vi "BMU诊断标定.vi"(8 "CAN端口":u16(ring), 9 "设备索引号":u16(ring), 10 "CAN卡类型":u32(ring)=21) -> ()   [LabVIEW 2013] (continued)
    tunnel: w59 -> [w3721]
    tunnel: [w3720] -> w63
    tunnel: [w3719] -> w62
    tunnel: w27 -> [_]
    tunnel: w22 -> [w3711]
    stop <- w3718 stop-if-true
    n2828 = local read "停止"() -> (w3718:bool)
    n2829 = local read "设备索引号"() -> (w3715:u16)
    n2830 = local read "CAN卡类型"() -> (w3716:u32)
    n2831 = local read "CAN端口"() -> (w3714:u16)
    n2832 = call "receiver-8.6.vi"("错误输入（无错误）"=w3711, "CAN端口"=w3714, "设备索引号"=w3715, "CAN卡类型"=w3716) -> ("错误输出"=w3717:errorcluster, "输出簇"=w3713:T25, "接收成功"=w3712:bool)  [unwired: 3 out]
    n2833 = call <vilib>:"Clear Errors.vi"("error in (no error)"=w3717) -> ()  [unwired: 6 in, 1 out]
    n2834 = case shown="真" w3712 {
      tunnel: w3721 -> [w3723 w3729]
      tunnel: w3713 -> [_ w3728]
      tunnel: w3722 -> [w3724 w3727]
      tunnel: [w3724 w3726] -> w3720
      tunnel: [w3723 w3725] -> w3719
      frame False {
      }
      frame True {
        n2835 = Enqueue Element(queue=w3727, element=w3728, error in (no error)=w3729) -> (queue out=w3726:refnum<queue>, error out=w3725:errorcluster)  [unwired: 2 out]
      }
    }
  }
  n2836 = while {
    tunnel: w60 -> [w3739]
    tunnel: w59 -> [w3738]
    tunnel: w8 -> [w3731]
    stop <- w3732 stop-if-true
    n2837 = global read "全局 1.vi" "名称"() -> (w3730:string)
    n2838 = local read "停止"() -> (w3732:bool)
    n2839 = local read "控制1"() -> (w3734:bool)
    n2840 = Dequeue Element(queue=w3739, timeout in ms (-1)=50 ("超时毫秒(-1)"), error in (no error)=w3738) -> (element=w3737:T3, error out=w3736:errorcluster)  [unwired: 2 out]
    n2841 = case shown="无错误" w3736 {
      tunnel: w3737 -> [w3746 _]
      tunnel: "写?" -> [w3743 _]
      tunnel: w3734 -> [w3742 _]
      tunnel: w3731 -> [w3741 _]
      tunnel: w3730 -> [w3740 _]
      frame No Error {
        n2842 = Unbundle(w3746) -> ("return type"=w3745:u32, "pReceive"=w3744:T26)
        n2843 = for {
          N: w3745 -> [_]
          tunnel: w3744 -> [w3752] mode=indexing
          tunnel: w3743 -> [w3750]
          tunnel: w3742 -> [w3749]
          tunnel: w3741 -> [w3748]
          tunnel: w3740 -> [w3747]
          n2844 = Unbundle By Name(w3752) -> ("ID"=w3753:u32)
          n2845 = call "ID解析.vi"("ID"=w3753) -> ("PDU(1)"=w3751:i32)  [unwired: 10 out]
          n2846 = case shown="18" w3751 {
            tunnel: w3752 -> [_ w3765]
            tunnel: w3750 -> [_ w3757]
            tunnel: w3749 -> [_ w3756]
            tunnel: w3748 -> [_ w3755]
            tunnel: w3747 -> [_ w3754]
            frame 0, Default {
            }
            frame 24 {
              n2847 = local read "主从选择"() -> (w3758:enum32{"主板", "从板"})
              n2848 = local read "设备索引号"() -> (w3761:u16)
              n2849 = local read "CAN卡类型"() -> (w3760:u32)
              n2850 = local read "CAN端口"() -> (w3762:u16)
              n2851 = case shown="\"从板\"" w3758 {
                tunnel: [0 ("FUNC") w3768] -> w3759
                tunnel: w3755 -> [_ w3769]
                tunnel: w3754 -> [_ w3767]
                frame "主板", Default {
                }
                frame "从板" {
                  n2852 = local read "从板号"() -> (w3770:u8)
                  n2853 = Equal?(x=w3767, y="从板号") -> (x = y?=w3771:bool)
                  n2854 = Select(t=w3769, s=w3771, f=w3770) -> (s? t:f=w3768:i32)
                }
              }
              n2855 = disable-structure shown="禁用" {
                disable-tunnel: w3765 -> [w3773 _]
                frame Disabled {
                  n2856 = call "标定授权读取.vi"("VCI_Receive"=w3773) -> ()  [unwired: 1 out]
                }
                frame Enabled {
                }
              }
              n2857 = local read "面板选择"() -> (w3764:T7)
              n2858 = case shown="\"读写参数\", 默认" w3764 {
                tunnel: w3757 -> [w3778 _ _ _]
                tunnel: "命令" -> [w3779 w3879 w4134 w4274]
                tunnel: w3758 -> [w3788 _ w4142 w4282]
                tunnel: w3765 -> [_ _ _ _]
                tunnel: w3765 -> [w3784 w3880 w4136 w4276]
                tunnel: w3762 -> [w3783 w3881 w4137 w4277]
                tunnel: w3761 -> [w3782 w3882 w4138 w4278]
                tunnel: w3760 -> [w3781 w3883 w4139 w4279]
                tunnel: w3759 -> [w3780 _ w4135 w4275]
                tunnel: w3756 -> [w3774 _ _ _]
                frame "读写参数", Default {
                  n2859 = local read "命令序号"() -> (w3777:u8)
                  n2860 = call "多帧接收机制(EV05).vi"("can卡类型"=w3781, "设备索引号"=w3782, "CAN端口"=w3783, "VCI_Receive"=w3784, "命令"=w3779, "板号"=w3780, "写?"=w3778, "命令序号"=w3777) -> ("错误信号"=w3775:bool, "错误代码"=w3787:i32, "输出数组"=w3786:u8[], "读错误代码"=w3776:u8[], "结束信号"=w3785:bool)  [unwired: 7 out]
                  n2861 = case shown="假" w3778 {
                    tunnel: w3785 -> [w3798 w3862]
                    tunnel: w3787 -> [w3797 w3861]
                    tunnel: w3777 -> [w3796 _]
                    tunnel: w3786 -> [w3795 _]
                    tunnel: w3779 -> [w3794 _]
                    tunnel: w3788 -> [w3792 w3860]
                    tunnel: w3776 -> [w3791 _]
                    tunnel: w3775 -> [w3790 _]
                    tunnel: w3774 -> [w3789 _]
                    frame False {
                      # "读参数"
                      n2862 = And(x=w3789, y=w3798) -> (x .and. y?=w3793:bool)
                      n2863 = case shown="真" w3793 {
                        tunnel: w3797 -> [_ w3809]
                        tunnel: w3796 -> [_ w3808]
                        tunnel: w3795 -> [_ w3807]
                        tunnel: w3794 -> [_ w3806]
                        tunnel: w3792 -> [_ w3802]
                        tunnel: w3791 -> [_ w3800]
                        tunnel: w3790 -> [_ w3801]
                        frame False {
                        }
                        frame True {
                          n2864 = case shown="假" w3801 {
                            tunnel: w3809 -> [w3819 _]
                            tunnel: w3808 -> [w3818 _]
                            tunnel: w3807 -> [w3817 _]
                            tunnel: w3806 -> [w3815 _]
                            tunnel: w3802 -> [w3811 _]
                            tunnel: w3800 -> [_ w3845]
                            frame False {
                              n2865 = case shown="\"从板\"" w3811 {
                                tunnel: [w3820 _] -> w3814
                                tunnel: [_ w3833] -> w3813
                                frame "主板", Default {
                                n2866 = stacked-sequence {
                                tunnel: [_ w3832] -> w3820
                                frame #0 {
                                n2867 = control-ref of="一级故障"() -> (w3826:refnum<vi>)
                                n2868 = control-ref of="一级故障 2"() -> (w3828:refnum<vi>)
                                n2869 = control-ref of="一级故障 3"() -> (w3829:refnum<vi>)
                                n2870 = control-ref of="加热控制参数"() -> (w3830:refnum<vi>)
                                n2871 = control-ref of="充电控制参数"() -> (w3831:refnum<vi>)
                                n2872 = control-ref of="电池信息"() -> (w3824:refnum<vi>)
                                n2873 = control-ref of="项目信息"() -> (w3827:refnum<vi>)
                                n2874 = control-ref of="项目信息2"() -> (w3825:refnum<vi>)
                                n2875 = control-ref of="高压参数"() -> (w3823:refnum<vi>)
                                n2876 = local read "主板数据"() -> (w3822:T4)
                                n2877 = Bundle(cluster=w3822, "项目信息"=w3827, "一级故障 4"=w3825, "一级故障"=w3826, "一级故障 2"=w3828, "一级故障 3"=w3829, "加热控制参数"=w3830, "充电控制参数"=w3831, "高压参数"=w3823, "电池信息"=w3824) -> (w3821:T4)
                                n2878 = local write "主板数据"(w3821) -> ()
                                }
                                frame #1 {
                                n2879 = control-ref of="主板数据"() -> (w3832:refnum<vi>)
                                }
                                }
                                }
                                frame "从板" {
                                n2880 = stacked-sequence {
                                tunnel: [_ w3844] -> w3833
                                frame #0 {
                                n2881 = control-ref of="从板号"() -> (w3838:refnum<vi>)
                                n2882 = control-ref of="项目信息 2"() -> (w3839:refnum<vi>)
                                n2883 = control-ref of="电池组信息"() -> (w3837:refnum<vi>)
                                n2884 = control-ref of="加热控制参数"() -> (w3840:refnum<vi>)
                                n2885 = control-ref of="一级故障(从板)"() -> (w3841:refnum<vi>)
                                n2886 = control-ref of="二级故障(从板)"() -> (w3842:refnum<vi>)
                                n2887 = control-ref of="三级故障(从板)"() -> (w3843:refnum<vi>)
                                n2888 = control-ref of="均衡参数"() -> (w3836:refnum<vi>)
                                n2889 = local read "从板信息"() -> (w3835:T2)
                                n2890 = Bundle(cluster=w3835, "从板号"=w3838, "项目信息 2"=w3839, "加热控制参数"=w3840, "一级故障(从板)"=w3841, "二级故障(从板)"=w3842, "三级故障(从板)"=w3843, "电池组信息(从板)"=w3837, "均衡参数"=w3836) -> (w3834:T2)
                                n2891 = local write "从板信息"(w3834) -> ()
                                }
                                frame #1 {
                                n2892 = control-ref of="从板信息"() -> (w3844:refnum<vi>)
                                }
                                }
                                }
                              }
                              n2893 = control-ref of="结果"() -> (w3816:refnum<vi>)
                              n2894 = control-ref of="从板个数"() -> (w3812:refnum<vi>)
                              n2895 = control-ref of="二维码"() -> (w3810:refnum<vi>)
                              n2896 = call "输出数据解析.vi"("主板引用"=w3814, "从板引用"=w3813, "板选择"=w3811, "错误代码"=w3819, "命令序号"=w3818, "输入数组"=w3817, "命令"=w3815, "进度引用"=w3816, "从板个数"=w3812, "从板二维码信息"=w3810) -> ()  [unwired: 1 in, 5 out]
                            }
                            frame True {
                              n2897 = Index Array(array=w3845, index #1=0 ("索引"), index #2=1 ("索引")) -> (element #1=w3848:u8, element #2=w3849:u8)
                              n2898 = Join Numbers(hi=w3848, lo=w3849) -> ((hi.lo)=w3847:u16)
                              n2899 = Number To Hexadecimal String(2:w3847) -> (0:w3846:string)  [unwired: 1 out]
                              n2900 = control-ref of="结果"() -> (w3854:refnum<vi>)
                              n2901 = Concatenate Strings("0x" ("字符串"), w3846) -> (w3855:string)
                              n2902 = Build Array(w3855) -> (w3856:string[])
                              n2903 = call "表格编辑.vi"("新元素/子数组"=w3856, "活动单元格:单元格背景色"=u32 16740749, "MCListbox引用句柄"=w3854) -> ()  [unwired: 9 out]
                            }
                          }
                          n2904 = global write "EV05全局变量1.vi" "流控帧 2"(FALSE ("流控帧 2")) -> ()
                          n2905 = global write "EV05全局变量1.vi" "输出数组"(i32[] []) -> ()
                          n2906 = local write "控制1"(FALSE ("控制1")) -> ()
                          n2907 = local write "消除"(FALSE ("消除")) -> ()
                        }
                      }
                    }
                    frame True {
                      # "写参数判定"
                      n2908 = And(x="控制1", y=w3862) -> (x .and. y?=w3859:bool)
                      n2909 = case shown="真" w3859 {
                        tunnel: w3861 -> [_ w3869]
                        tunnel: w3860 -> [_ w3866]
                        frame False {
                        }
                        frame True {
                          n2910 = call <vilib>:"Unset Busy.vi"() -> ()  [unwired: 2 in, 10 out]
                          n2911 = case shown="\"从板\"" w3866 {
                            tunnel: [w3870 w3871] -> w3868
                            frame "主板", Default {
                              n2912 = local read "主板选项"() -> (w3870:string)
                            }
                            frame "从板" {
                              n2913 = local read "从板选项"() -> (w3871:string)
                            }
                          }
                          n2914 = control-ref of="结果"() -> (w3867:refnum<vi>)
                          n2915 = call "输入数据判定.vi"("主从选择"=w3866, "主板选项"=w3868, "进度引用"=w3867, "错误代码"=w3869) -> ()  [unwired: 2 in, 6 out]
                          n2916 = global write "EV05全局变量1.vi" "流控帧 2"(FALSE ("流控帧 2")) -> ()
                          n2917 = local write "控制1"(FALSE ("控制1")) -> ()
                          n2918 = local write "消除"(FALSE ("消除")) -> ()
                        }
                      }
                      n2919 = global write "EV05全局变量1.vi" "输出数组"(i32[] []) -> ()
                    }
                  }
                }
                frame "版本读取" {
                  n2920 = local read "命令序号"() -> (w3872:u8)
                  n2921 = local read "从板板号"() -> (w3875:u8)
                  n2922 = local read "控制1"() -> (w3876:bool)
                  n2923 = call "多帧接收机制(EV05).vi"("can卡类型"=w3883, "设备索引号"=w3882, "CAN端口"=w3881, "VCI_Receive"=w3880, "命令"=w3879, "板号"=w3875, "命令序号"=w3872) -> ("错误信号"=w3873:bool, "输出数组"=w3884:u8[], "读错误代码"=w3874:u8[], "结束信号"=w3878:bool)  [unwired: 1 in, 8 out]
                  n2924 = And(x=w3876, y=w3878) -> (x .and. y?=w3877:bool)
                  n2925 = case shown="真" w3877 {
                    tunnel: w3884 -> [_ w3892]
                    tunnel: w3872 -> [_ w3891]
                    tunnel: w3879 -> [_ w3890]
                    tunnel: w3874 -> [_ w3886]
                    tunnel: w3873 -> [_ w3885]
                    frame False {
                    }
                    frame True {
                      n2926 = case shown="假" w3885 {
                        tunnel: w3892 -> [w3896 _]
                        tunnel: w3891 -> [w3895 _]
                        tunnel: w3890 -> [w3894 _]
                        tunnel: w3886 -> [w3893 w4120]
                        frame False {
                          n2927 = case shown="89" w3894 {
                            tunnel: w3895 -> [_ w3899]
                            tunnel: w3896 -> [_ w3898]
                            tunnel: w3893 -> [_ _]
                            frame 0, Default {
                            }
                            frame 137 {
                              n2928 = case shown="1" w3899 {
                                tunnel: w3898 -> [_ w3927 w3971 w3991 w4118]
                                frame 0, Default {
                                }
                                frame 1 {
                                w3909 = "." ("字符串")
                                n2929 = Array Subset(array=w3927, index=0 ("索引"), length=14 ("长度")) -> (w3940:u8[])
                                n2930 = Index Array(array=w3927, index=14 ("索引")) -> (element=w3930:u8)
                                n2931 = Index Array(array=w3927, index #1=15 ("索引"), index #2=16 ("索引")) -> (element #1=w3936:u8, element #2=w3937:u8)
                                n2932 = Index Array(array=w3927, index #1=17 ("索引"), index #2=18 ("索引")) -> (element #1=w3931:u8, element #2=w3932:u8)
                                n2933 = call "数组去零.vi"("输入"=w3940) -> ("输出"=w3915:dbl[])
                                n2934 = Join Numbers(hi=w3931, lo=w3932) -> ((hi.lo)=w3928:u16)
                                n2935 = Join Numbers(hi=w3936, lo=w3937) -> ((hi.lo)=w3929:u16)
                                n2936 = Number To Decimal String(number=w3930) -> (decimal integer string=w3922:string)  [unwired: 1 out]
                                n2937 = Byte Array To String(unsigned byte array=w3915) -> (string=w3914:string)
                                n2938 = Number To Decimal String(number=w3928) -> (decimal integer string=w3910:string)  [unwired: 1 out]
                                n2939 = Number To Decimal String(number=w3929) -> (decimal integer string=w3921:string)  [unwired: 1 out]
                                n2940 = Array Subset(array=w3927, index=21 ("索引"), length=7 ("长度")) -> (w3924:u8[])
                                n2941 = Concatenate Strings("V" ("字符串"), w3922, w3909, w3921, w3909, w3910) -> (w3919:string)
                                n2942 = call "数组去零.vi"("输入"=w3924) -> ("输出"=w3907:dbl[])
                                n2943 = Byte Array To String(unsigned byte array=w3907) -> (string=w3905:string)
                                n2944 = call <vilib>:"Space Constant.vi"() -> ("String"=w3906:string)
                                n2945 = Equal?(x=w3905, y=w3906) -> (x = y?=w3911:bool)
                                n2946 = Concatenate Strings("-" ("字符串"), w3905) -> (w3912:string)
                                n2947 = Select(t=w3906, s=w3911, f=w3912) -> (s? t:f=w3908:string)
                                n2948 = Concatenate Strings(w3914, "-" ("字符串"), w3919, w3908) -> (w3901:string)
                                n2949 = local read "项目软件版本"() -> (w3903:string[])
                                n2950 = local read "从板板号"() -> (w3900:u8)
                                n2951 = local write "项目软件版本号"(w3901) -> ()
                                n2952 = Replace Array Subset(array=w3903, new element=w3901, index=w3900) -> (w3902:string[])
                                n2953 = control-ref of="结果"() -> (w3918:refnum<vi>)
                                n2954 = local write "项目软件版本"(w3902) -> ()
                                n2955 = Build Array("项目软件版本     读取完成" ("读取结果")) -> (w3916:string[])
                                n2956 = call "表格编辑(版本读取).vi"("新元素/子数组"=w3916, "活动单元格:单元格背景色"=u32 6618880, "MCListbox引用句柄"=w3918) -> ()  [unwired: 9 out]
                                }
                                frame 2 {
                                w3954 = ""
                                w3951 = "." ("字符串")
                                n2957 = Array Subset(array=w3971, index=0 ("索引"), length=14 ("长度")) -> (w3959:u8[])
                                n2958 = Index Array(array=w3971, index=14 ("索引")) -> (element=w3974:u8)
                                n2959 = Index Array(array=w3971, index #1=15 ("索引"), index #2=16 ("索引")) -> (element #1=w3980:u8, element #2=w3981:u8)
                                n2960 = Index Array(array=w3971, index #1=17 ("索引"), index #2=18 ("索引")) -> (element #1=w3975:u8, element #2=w3976:u8)
                                n2961 = Join Numbers(hi=w3975, lo=w3976) -> ((hi.lo)=w3972:u16)
                                n2962 = Join Numbers(hi=w3980, lo=w3981) -> ((hi.lo)=w3973:u16)
                                n2963 = Number To Decimal String(number=w3972) -> (decimal integer string=w3952:string)  [unwired: 1 out]
                                n2964 = call "数组去零.vi"("输入"=w3959) -> ("输出"=w3958:dbl[])
                                n2965 = Number To Decimal String(number=w3974) -> (decimal integer string=w3966:string)  [unwired: 1 out]
                                n2966 = Number To Decimal String(number=w3973) -> (decimal integer string=w3965:string)  [unwired: 1 out]
                                n2967 = Array Subset(array=w3971, index=21 ("索引"), length=7 ("长度")) -> (w3968:u8[])
                                n2968 = Byte Array To String(unsigned byte array=w3958) -> (string=w3953:string)
                                n2969 = call "数组去零.vi"("输入"=w3968) -> ("输出"=w3950:dbl[])
                                n2970 = Concatenate Strings("V" ("字符串"), w3966, w3951, w3965, w3951, w3952) -> (w3963:string)
                                n2971 = Byte Array To String(unsigned byte array=w3950) -> (string=w3948:string)
                                n2972 = Equal?(x=w3954, y=w3948) -> (x = y?=w3955:bool)
                                n2973 = Concatenate Strings("-" ("字符串"), w3948) -> (w3956:string)
                                n2974 = Select(t=w3954, s=w3955, f=w3956) -> (s? t:f=w3949:string)
                                n2975 = Concatenate Strings(w3953, "-" ("字符串"), w3963, w3949) -> (w3944:string)
                                n2976 = local read "平台软件版本"() -> (w3946:string[])
                                n2977 = local read "从板板号"() -> (w3943:u8)
                                n2978 = local write "平台软件版本号"(w3944) -> ()
                                n2979 = Replace Array Subset(array=w3946, new element=w3944, index=w3943) -> (w3945:string[])
                                n2980 = control-ref of="结果"() -> (w3961:refnum<vi>)
                                n2981 = local write "平台软件版本"(w3945) -> ()
                                n2982 = Build Array("平台软件版本     读取完成" ("读取结果")) -> (w3960:string[])
                                n2983 = call "表格编辑(版本读取).vi"("新元素/子数组"=w3960, "活动单元格:单元格背景色"=u32 6618880, "MCListbox引用句柄"=w3961) -> ()  [unwired: 1 in, 8 out]
                                }
                                frame 3 {
                                n2984 = Index Array(array=w3991, index #1=0 ("索引"), index #2=1 ("索引")) -> (element #1=w3987:u8, element #2=w3988:u8)
                                n2985 = Join Numbers(hi=w3987, lo=w3988) -> ((hi.lo)=w3986:u16)
                                n2986 = case shown="99, 默认" w3986 {
                                tunnel: w3991 -> [w3994 _ w4028]
                                tunnel: w3986 -> [_ _ w4006]
                                frame 0 {
                                n2987 = Index Array(array=w3994, index #1=2 ("索引"), index #2=3 ("索引")) -> (element #1=w3998:u8, element #2=w3997:u8)
                                n2988 = Join Numbers(hi=w3998, lo=w3997) -> ((hi.lo)=w3993:u16)
                                n2989 = for {
                                N: w3993 -> [_]
                                tunnel: w3994 -> [w4003]
                                tunnel: [w3999] -> w3992 mode=indexing
                                i -> [w4002]
                                n2990 = Add(x=w4002, y=4) -> (x+y=w4000:i32)
                                n2991 = Index Array(array=w4003, index=w4000) -> (element=w3999:u8)
                                }
                                "MODEL号" <- w3992
                                }
                                frame 99, Default {
                                }
                                frame 1..40 {
                                w4011 = ""
                                w4032 = "." ("字符串")
                                n2992 = Array Subset(array=w4028, index=2 ("索引"), length=14 ("长度")) -> (w4017:u8[])
                                n2993 = Index Array(array=w4028, index=16 ("索引")) -> (element=w4040:u8)
                                n2994 = Index Array(array=w4028, index #1=17 ("索引"), index #2=18 ("索引")) -> (element #1=w4046:u8, element #2=w4047:u8)
                                n2995 = Index Array(array=w4028, index #1=19 ("索引"), index #2=20 ("索引")) -> (element #1=w4041:u8, element #2=w4042:u8)
                                n2996 = Join Numbers(hi=w4041, lo=w4042) -> ((hi.lo)=w4038:u16)
                                n2997 = Join Numbers(hi=w4046, lo=w4047) -> ((hi.lo)=w4039:u16)
                                n2998 = Number To Decimal String(number=w4006) -> (decimal integer string=w4026:string)  [unwired: 1 out]
                                n2999 = Number To Decimal String(number=w4040) -> (decimal integer string=w4034:string)  [unwired: 1 out]
                                n3000 = call "数组去零.vi"("输入"=w4017) -> ("输出"=w4016:dbl[])
                                n3001 = Number To Decimal String(number=w4039) -> (decimal integer string=w4033:string)  [unwired: 1 out]
                                n3002 = Number To Decimal String(number=w4038) -> (decimal integer string=w4031:string)  [unwired: 1 out]
                                n3003 = Byte Array To String(unsigned byte array=w4016) -> (string=w4018:string)
                                n3004 = Concatenate Strings("第" ("读取结果"), w4026, "模块" ("字符串"), "     读取完成" ("读取结果")) -> (w4019:string)
                                n3005 = Concatenate Strings("V" ("字符串"), w4034, w4032, w4033, w4032, w4031) -> (w4029:string)
                                n3006 = control-ref of="结果"() -> (w4022:refnum<vi>)
                                n3007 = Array Subset(array=w4028, index=23 ("索引"), length=7 ("长度")) -> (w4015:u8[])
                                n3008 = call "数组去零.vi"("输入"=w4015) -> ("输出"=w4010:dbl[])
                                n3009 = Byte Array To String(unsigned byte array=w4010) -> (string=w4007:string)
                                n3010 = Build Array(w4019) -> (w4021:string[])
                                n3011 = control-ref of="模块软件版本 2"() -> (w4023:refnum<vi>)
                                n3012 = local read "模块软件版本"() -> (w4024:T1)
                                n3013 = Equal?(x=w4011, y=w4007) -> (x = y?=w4012:bool)
                                n3014 = call "表格编辑(版本读取).vi"("新元素/子数组"=w4021, "活动单元格:单元格背景色"=u32 6618880, "MCListbox引用句柄"=w4022) -> ()  [unwired: 1 in, 8 out]
                                n3015 = Concatenate Strings("-" ("字符串"), w4007) -> (w4013:string)
                                n3016 = Select(t=w4011, s=w4012, f=w4013) -> (s? t:f=w4009:string)
                                n3017 = Concatenate Strings(w4018, "-" ("字符串"), w4029, w4009) -> (w4008:string)
                                n3018 = case shown="30" w4006 {
                                tunnel: [_ "VERSIONM" "BCUMCAL" "BMUMCAL" "BMURMCAL" "BCUCMCAL" "BCUDMCAL" "SCH" "BSW" "CDD" "DATALAYER" "DATAANALYSIS" "SOC" "SOH" "SOF" "INTRES" "INTCAN" "CARCAN" "CHGCANL" "THM" "CHGM" "HVM" "LVM" "BALM" "SAFEM" "RUNMODEM" "RELAY" "DO" "GBCHGDET" "SUPPLYPOWGDET" "SUMVDET" "CURDET" "TEMPERDET" "CELLVDET" "ISODET" "AI" "DI" "SYSCONF" "ECUCONF"] -> w4005
                                frame 0, Default {
                                }
                                frame 1 {
                                }
                                frame 2 {
                                }
                                frame 3 {
                                }
                                frame 4 {
                                }
                                frame 5 {
                                }
                                frame 6 {
                                }
                                frame 7 {
                                }
                                frame 8 {
                                }
                                frame 9 {
                                }
                                frame 10 {
                                }
                                frame 11 {
                                }
                                frame 12 {
                                }
                                frame 13 {
                                }
                                frame 14 {
                                }
                                frame 15 {
                                }
                                frame 16 {
                                }
                                frame 17 {
                                }
                                frame 18 {
                                }
                                frame 19 {
                                }
                                frame 20 {
                                }
                                frame 21 {
                                }
                                frame 22 {
                                }
                                frame 23 {
                                }
                                frame 24 {
                                }
                                frame 25 {
                                }
                                frame 26 {
                                }
                                frame 27 {
                                }
                                frame 28 {
                                }
                                frame 29 {
                                }
                                frame 30 {
                                }
                                frame 31 {
                                }
                                frame 32 {
                                }
                                frame 33 {
                                }
                                frame 34 {
                                }
                                frame 35 {
                                }
                                frame 36 {
                                }
                                frame 37 {
                                }
                                frame 38 {
                                }
                                }
                                n3019 = case shown="\"全部读取\"" w4024 {
                                tunnel: w4008 -> [w4091 w4099]
                                tunnel: w4006 -> [w4095 w4104]
                                tunnel: w4023 -> [w4097 w4105]
                                tunnel: w4005 -> [w4096 w4103]
                                frame "全部读取" {
                                n3020 = Number To Decimal String(number=w4095) -> (decimal integer string=w4094:string)  [unwired: 1 out]
                                n3021 = Concatenate Strings(w4094, "-" ("元素"), w4096) -> (w4092:string)
                                n3022 = Build Array(w4092, w4091) -> (w4090:string[])
                                n3023 = call "表格编辑(模块版本).vi"("新元素/子数组"=w4090, "MCListbox引用句柄"=w4097) -> ()  [unwired: 1 in, 9 out]
                                }
                                frame "BCUMCAL", Default {
                                n3024 = Number To Decimal String(number=w4104) -> (decimal integer string=w4102:string)  [unwired: 1 out]
                                n3025 = Concatenate Strings(w4102, "-" ("元素"), w4103) -> (w4100:string)
                                n3026 = Build Array(w4100, w4099) -> (w4098:string[])
                                n3027 = call "表格编辑(模块版本).vi"("新元素/子数组"=w4098, "MCListbox引用句柄"=w4105) -> ()  [unwired: 1 in, 9 out]
                                }
                                }
                                }
                                }
                                }
                                frame 4 {
                                n3028 = Array Subset(array=w4118, length=12 ("长度")) -> (w4116:u8[])  [unwired: 1 in]
                                n3029 = Byte Array To String(unsigned byte array=w4116) -> (string=w4115:string)
                                n3030 = call <vilib>:"Trim Whitespace.vi"("string"=w4115) -> ("trimmed string"=w4107:string)  [unwired: 1 in]
                                n3031 = local read "从板板号"() -> (w4106:u8)
                                n3032 = local write "硬件版本号"(w4107) -> ()
                                n3033 = local read "硬件版本"() -> (w4108:string[])
                                n3034 = Replace Array Subset(array=w4108, new element=w4107, index=w4106) -> (w4109:string[])
                                n3035 = local write "硬件版本"(w4109) -> ()
                                n3036 = global write "EV05全局变量1.vi" "写入超时"(TRUE ("写入超时")) -> ()
                                n3037 = control-ref of="结果"() -> (w4113:refnum<vi>)
                                n3038 = Build Array("硬件版本     读取完成" ("读取结果")) -> (w4112:string[])
                                n3039 = call "表格编辑(版本读取).vi"("新元素/子数组"=w4112, "活动单元格:单元格背景色"=u32 6618880, "MCListbox引用句柄"=w4113) -> ()  [unwired: 9 out]
                                }
                              }
                              n3040 = global write "EV05全局变量1.vi" "写入超时"(TRUE ("写入超时")) -> ()
                            }
                          }
                        }
                        frame True {
                          n3041 = Index Array(array=w4120, index #1=0 ("索引"), index #2=1 ("索引")) -> (element #1=w4125:u8, element #2=w4126:u8)
                          n3042 = Join Numbers(hi=w4125, lo=w4126) -> ((hi.lo)=w4124:u16)
                          n3043 = Number To Hexadecimal String(2:w4124) -> (0:w4123:string)  [unwired: 1 out]
                          n3044 = control-ref of="结果"() -> (w4122:refnum<vi>)
                          n3045 = Concatenate Strings("0x" ("字符串"), w4123) -> (w4130:string)
                          n3046 = Build Array(w4130) -> (w4121:string[])
                          n3047 = call "表格编辑(版本读取).vi"("新元素/子数组"=w4121, "活动单元格:单元格背景色"=u32 16740749, "MCListbox引用句柄"=w4122) -> ()  [unwired: 9 out]
                        }
                      }
                      n3048 = global write "EV05全局变量1.vi" "流控帧 2"(FALSE ("流控帧 2")) -> ()
                      n3049 = local write "控制1"(FALSE ("控制1")) -> ()
                      n3050 = local write "消除"(FALSE ("消除")) -> ()
                      n3051 = call <vilib>:"Unset Busy.vi"() -> ()  [unwired: 2 in, 10 out]
                    }
                  }
                }
                frame "其它诊断" {
                  n3052 = local read "命令序号"() -> (w4132:u8)
                  n3053 = call "多帧接收机制(EV05).vi"("can卡类型"=w4139, "设备索引号"=w4138, "CAN端口"=w4137, "VCI_Receive"=w4136, "命令"=w4134, "板号"=w4135, "命令序号"=w4132) -> ("错误代码"=w4141:i32, "输出数组"=w4133:u8[], "读错误代码"=w4131:u8[], "结束信号"=w4140:bool)  [unwired: 1 in, 8 out]
                  n3054 = case shown="真" w4140 {
                    tunnel: w4142 -> [_ w4143]
                    tunnel: w4141 -> [_ _]
                    tunnel: w4133 -> [_ w4144]
                    tunnel: w4132 -> [_ w4147]
                    tunnel: w4131 -> [_ w4145]
                    frame False {
                    }
                    frame True {
                      n3055 = Insert Into Array(array=w4145, new element=w4144) -> (w4146:u8[])  [unwired: 1 in]
                      n3056 = case shown="1" w4147 {
                        tunnel: w4146 -> [_ w4156 w4242]
                        tunnel: w4143 -> [_ _ w4237]
                        frame 0, Default {
                        }
                        frame 1 {
                          n3057 = Index Array(array=w4156) -> (element #1=w4155:u8, element #2=w4154:u8, element #3=w4153:u8)  [unwired: 3 in]
                          n3058 = Join Numbers(hi=w4154, lo=w4153) -> ((hi.lo)=w4152:u16)
                          n3059 = case shown="4" w4155 {
                            tunnel: w4156 -> [_ _ _ _ _ _ _ _ _ _]
                            tunnel: w4152 -> [_ w4159 w4167 w4177 w4187 w4197 w4207 w4217 w4227 _]
                            frame 0, Default {
                              n3060 = local write "继电器超时处理"(FALSE ("继电器超时处理")) -> ()
                            }
                            frame 1 {
                              n3061 = Equal To 0?(x=w4159) -> (x = 0?=w4158:bool)
                              n3062 = local write "正级继电器 12"(w4158) -> ()
                              n3063 = case shown="假" w4158 {
                                tunnel: w4159 -> [w4162 _]
                                frame False {
                                n3064 = local read "正级继电器"() -> (w4164:bool)
                                n3065 = Number To Hexadecimal String(2:w4162) -> (0:w4161:string)  [unwired: 1 out]
                                n3066 = local write "继电器超时处理"(TRUE ("继电器超时处理")) -> ()
                                n3067 = Not(x=w4164) -> (.not. x?=w4163:bool)
                                n3068 = Concatenate Strings("继电器操作失败,0x" ("消息"), w4161) -> ()  [unwired: 1 out]
                                n3069 = local write "正级继电器"(w4163) -> ()
                                }
                                frame True {
                                (unwired) "继电器操作成功!\n继电器操作成功!\n继电器操作成功!"
                                }
                              }
                            }
                            frame 2 {
                              n3070 = Equal To 0?(x=w4167) -> (x = 0?=w4166:bool)
                              n3071 = case shown="假" w4166 {
                                tunnel: w4167 -> [w4173 _]
                                tunnel: [w4171 "继电器操作成功!\n继电器操作成功!\n继电器操作成功!"] -> _
                                frame False {
                                n3072 = local read "负级继电器"() -> (w4169:bool)
                                n3073 = Number To Hexadecimal String(2:w4173) -> (0:w4172:string)  [unwired: 1 out]
                                n3074 = local write "继电器超时处理"(TRUE ("继电器超时处理")) -> ()
                                n3075 = Not(x=w4169) -> (.not. x?=w4170:bool)
                                n3076 = Concatenate Strings("继电器操作失败,0x" ("消息"), w4172) -> (w4171:string)
                                n3077 = local write "负级继电器"(w4170) -> ()
                                }
                                frame True {
                                }
                              }
                              n3078 = local write "正级继电器 2"(w4166) -> ()
                            }
                            frame 3 {
                              n3079 = Equal To 0?(x=w4177) -> (x = 0?=w4176:bool)
                              n3080 = case shown="假" w4176 {
                                tunnel: w4177 -> [w4183 _]
                                tunnel: [w4181 "继电器操作成功!\n继电器操作成功!\n继电器操作成功!"] -> _
                                frame False {
                                n3081 = local read "预充电继电器"() -> (w4179:bool)
                                n3082 = Number To Hexadecimal String(2:w4183) -> (0:w4182:string)  [unwired: 1 out]
                                n3083 = local write "继电器超时处理"(TRUE ("继电器超时处理")) -> ()
                                n3084 = Not(x=w4179) -> (.not. x?=w4180:bool)
                                n3085 = Concatenate Strings("继电器操作失败,0x" ("消息"), w4182) -> (w4181:string)
                                n3086 = local write "预充电继电器"(w4180) -> ()
                                }
                                frame True {
                                }
                              }
                              n3087 = local write "正级继电器 3"(w4176) -> ()
                            }
                            frame 4 {
                              n3088 = Equal To 0?(x=w4187) -> (x = 0?=w4186:bool)
                              n3089 = case shown="假" w4186 {
                                tunnel: w4187 -> [w4193 _]
                                tunnel: [w4191 "继电器操作成功!\n继电器操作成功!\n继电器操作成功!"] -> _
                                frame False {
                                n3090 = local read "加热继电器"() -> (w4190:bool)
                                n3091 = Number To Hexadecimal String(2:w4193) -> (0:w4192:string)  [unwired: 1 out]
                                n3092 = local write "继电器超时处理"(TRUE ("继电器超时处理")) -> ()
                                n3093 = Not(x=w4190) -> (.not. x?=w4189:bool)
                                n3094 = Concatenate Strings("继电器操作失败,0x" ("消息"), w4192) -> (w4191:string)
                                n3095 = local write "加热继电器"(w4189) -> ()
                                }
                                frame True {
                                }
                              }
                              n3096 = local write "正级继电器 5"(w4186) -> ()
                            }
                            frame 5 {
                              n3097 = Equal To 0?(x=w4197) -> (x = 0?=w4196:bool)
                              n3098 = case shown="假" w4196 {
                                tunnel: w4197 -> [w4203 _]
                                tunnel: [w4201 "继电器操作成功!\n继电器操作成功!\n继电器操作成功!"] -> _
                                frame False {
                                n3099 = local read "充电继电器"() -> (w4199:bool)
                                n3100 = Number To Hexadecimal String(2:w4203) -> (0:w4202:string)  [unwired: 1 out]
                                n3101 = local write "继电器超时处理"(TRUE ("继电器超时处理")) -> ()
                                n3102 = Not(x=w4199) -> (.not. x?=w4200:bool)
                                n3103 = Concatenate Strings("继电器操作失败,0x" ("消息"), w4202) -> (w4201:string)
                                n3104 = local write "充电继电器"(w4200) -> ()
                                }
                                frame True {
                                }
                              }
                              n3105 = local write "正级继电器 4"(w4196) -> ()
                            }
                            frame 6 {
                              n3106 = Equal To 0?(x=w4207) -> (x = 0?=w4206:bool)
                              n3107 = local write "正级继电器 6"(w4206) -> ()
                              n3108 = case shown="假" w4206 {
                                tunnel: w4207 -> [w4213 _]
                                tunnel: [w4211 "继电器操作成功!\n继电器操作成功!\n继电器操作成功!"] -> _
                                frame False {
                                n3109 = local read "风机继电器"() -> (w4209:bool)
                                n3110 = Number To Hexadecimal String(2:w4213) -> (0:w4212:string)  [unwired: 1 out]
                                n3111 = local write "继电器超时处理"(TRUE ("继电器超时处理")) -> ()
                                n3112 = Not(x=w4209) -> (.not. x?=w4210:bool)
                                n3113 = Concatenate Strings("继电器操作失败,0x" ("消息"), w4212) -> (w4211:string)
                                n3114 = local write "风机继电器"(w4210) -> ()
                                }
                                frame True {
                                }
                              }
                            }
                            frame 7 {
                              n3115 = Equal To 0?(x=w4217) -> (x = 0?=w4216:bool)
                              n3116 = case shown="假" w4216 {
                                tunnel: w4217 -> [w4222 _]
                                tunnel: [w4220 "继电器操作成功!\n继电器操作成功!\n继电器操作成功!"] -> _
                                frame False {
                                n3117 = local read "加热继电器(从)"() -> (w4218:bool)
                                n3118 = Number To Hexadecimal String(2:w4222) -> (0:w4221:string)  [unwired: 1 out]
                                n3119 = Not(x=w4218) -> (.not. x?=w4219:bool)
                                n3120 = Concatenate Strings("继电器操作失败,0x" ("消息"), w4221) -> (w4220:string)
                                n3121 = local write "加热继电器(从)"(w4219) -> ()
                                }
                                frame True {
                                n3122 = local write "继电器超时处理"(TRUE ("继电器超时处理")) -> ()
                                }
                              }
                              n3123 = local write "正级继电器 7"(w4216) -> ()
                            }
                            frame 8 {
                              n3124 = Equal To 0?(x=w4227) -> (x = 0?=w4226:bool)
                              n3125 = case shown="假" w4226 {
                                tunnel: w4227 -> [w4232 _]
                                tunnel: [w4230 "继电器操作成功!\n继电器操作成功!\n继电器操作成功!"] -> _
                                frame False {
                                n3126 = local read "风机继电器(从)"() -> (w4228:bool)
                                n3127 = Number To Hexadecimal String(2:w4232) -> (0:w4231:string)  [unwired: 1 out]
                                n3128 = Not(x=w4228) -> (.not. x?=w4229:bool)
                                n3129 = Concatenate Strings("继电器操作失败,0x" ("消息"), w4231) -> (w4230:string)
                                n3130 = local write "风机继电器(从)"(w4229) -> ()
                                }
                                frame True {
                                n3131 = local write "继电器超时处理"(TRUE ("继电器超时处理")) -> ()
                                }
                              }
                              n3132 = local write "正级继电器 8"(w4226) -> ()
                            }
                            frame 85, 170 {
                              n3133 = local write "继电器超时处理"(TRUE ("继电器超时处理")) -> ()
                            }
                          }
                        }
                        frame 2 {
                          n3134 = Index Array(array=w4242) -> (element #1=w4241:u8, element #2=w4240:u8, element #3=w4239:u8)  [unwired: 3 in]
                          n3135 = Join Numbers(hi=w4240, lo=w4239) -> ((hi.lo)=w4238:u16)
                          n3136 = case shown="2" w4241 {
                            tunnel: w4242 -> [_ _ _]
                            tunnel: w4238 -> [_ w4246 w4260]
                            tunnel: w4237 -> [_ w4245 _]
                            frame 0, Default {
                              n3137 = local write "继电器超时处理"(FALSE ("继电器超时处理")) -> ()
                            }
                            frame 1 {
                              n3138 = Equal To 0?(x=w4246) -> (x = 0?=w4244:bool)
                              n3139 = case shown="假" w4244 {
                                tunnel: w4246 -> [w4252 _]
                                tunnel: [w4250 "DO控制操作成功!\nDO控制操作成功!\nDO控制操作成功!"] -> _
                                tunnel: w4245 -> [w4249 _]
                                frame False {
                                n3140 = case shown="\"主板\", 默认" w4249 {
                                frame "主板", Default {
                                n3141 = local read "DO1"() -> (w4255:bool)
                                n3142 = Not(x=w4255) -> (.not. x?=w4254:bool)
                                n3143 = local write "DO1"(w4254) -> ()
                                }
                                frame "从板" {
                                n3144 = local read "DO1 2"() -> (w4257:bool)
                                n3145 = Not(x=w4257) -> (.not. x?=w4256:bool)
                                n3146 = local write "DO1 2"(w4256) -> ()
                                }
                                }
                                n3147 = Number To Hexadecimal String(2:w4252) -> (0:w4251:string)  [unwired: 1 out]
                                n3148 = Concatenate Strings("DO控制操作失败,0x" ("消息"), w4251) -> (w4250:string)
                                }
                                frame True {
                                }
                              }
                              n3149 = case shown="\"从板\"" w4245 {
                                tunnel: w4244 -> [w4247 w4248]
                                frame "主板", Default {
                                n3150 = local write "正级继电器 9"(w4247) -> ()
                                }
                                frame "从板" {
                                n3151 = local write "正级继电器 11"(w4248) -> ()
                                }
                              }
                            }
                            frame 2 {
                              n3152 = Equal To 0?(x=w4260) -> (x = 0?=w4259:bool)
                              n3153 = case shown="假" w4259 {
                                tunnel: w4260 -> [w4265 _]
                                tunnel: [w4263 "DO控制操作成功!\nDO控制操作成功!\nDO控制操作成功!"] -> _
                                frame False {
                                n3154 = Number To Hexadecimal String(2:w4265) -> (0:w4264:string)  [unwired: 1 out]
                                n3155 = local read "DO2"() -> (w4262:bool)
                                n3156 = Not(x=w4262) -> (.not. x?=w4261:bool)
                                n3157 = Concatenate Strings("DO控制操作失败,0x" ("消息"), w4264) -> (w4263:string)
                                n3158 = local write "DO2"(w4261) -> ()
                                }
                                frame True {
                                }
                              }
                              n3159 = local write "正级继电器 10"(w4259) -> ()
                            }
                          }
                        }
                      }
                      n3160 = local write "消除"(FALSE ("消除")) -> ()
                      n3161 = global write "EV05全局变量1.vi" "流控帧 2"(FALSE ("流控帧 2")) -> ()
                      n3162 = local write "控制1"(FALSE ("控制1")) -> ()
                      "继电器超时处理" <- TRUE ("控制1")
                    }
                  }
                }
                frame "高压板校正" {
                  n3163 = local read "命令序号"() -> (w4272:u8)
                  n3164 = call "多帧接收机制(EV05).vi"("can卡类型"=w4279, "设备索引号"=w4278, "CAN端口"=w4277, "VCI_Receive"=w4276, "命令"=w4274, "板号"=w4275, "命令序号"=w4272) -> ("错误信号"=w4268:bool, "错误代码"=w4281:i32, "输出数组"=w4273:u8[], "读错误代码"=w4271:u8[], "结束信号"=w4280:bool)  [unwired: 1 in, 7 out]
                  n3165 = local read "控制1"() -> (w4269:bool)
                  n3166 = And(x=w4269, y=w4280) -> (x .and. y?=w4270:bool)
                  n3167 = case shown="真" w4270 {
                    tunnel: w4282 -> [_ w4286]
                    tunnel: w4281 -> [_ _]
                    tunnel: w4273 -> [_ w4284]
                    tunnel: w4272 -> [_ w4285]
                    tunnel: w4271 -> [_ w4287]
                    tunnel: w4268 -> [_ w4288]
                    frame False {
                    }
                    frame True {
                      n3168 = case shown="假" w4288 {
                        tunnel: w4287 -> [_ w4498]
                        tunnel: w4286 -> [_ _]
                        tunnel: w4285 -> [w4293 _]
                        tunnel: w4284 -> [w4292 _]
                        frame False {
                          n3169 = case shown="2" w4293 {
                            tunnel: w4292 -> [_ w4298 w4332 w4362 w4389 w4416 w4443 w4470]
                            frame 0, Default {
                            }
                            frame 1 {
                              n3170 = for {
                                N: 10 -> [_]
                                tunnel: w4298 -> [w4315]
                                shift-right: [w4302] -> w4296
                                shift-left: string[] [] -> [w4304]
                                i -> [w4301]
                                w4309 = 8 ("索引")
                                w4313 = 2 ("y")
                                n3171 = Multiply(x=w4301, y=w4313) -> (x*y=w4314:i32)
                                n3172 = Array Subset(array=w4315, index=w4314, length=w4313) -> (w4312:u8[])
                                n3173 = Index Array(array=w4312) -> (element #1=w4311:u8, element #2=w4310:u8)  [unwired: 2 in]
                                n3174 = call "二进制解析-8.6.vi"("索引"=w4309, "数值"=w4311) -> ("低位子数组"=w4308:i32[])  [unwired: 1 in, 2 out]
                                n3175 = call "二进制解析-8.6.vi"("索引"=w4309, "数值"=w4310) -> ("低位子数组"=w4307:i32[])  [unwired: 1 in, 2 out]
                                n3176 = Insert Into Array(array=w4308, new element=w4307) -> (w4306:i32[])  [unwired: 1 in]
                                n3177 = case shown="2" w4301 {
                                tunnel: [6 15 9 4 2 0 2] -> w4300
                                frame 0, Default {
                                }
                                frame 1 {
                                }
                                frame 2 {
                                }
                                frame 3..5 {
                                }
                                frame 8, 9 {
                                }
                                frame 7 {
                                }
                                frame 6 {
                                }
                                }
                                n3178 = Reverse 1D Array(array=w4306) -> (reversed array=w4305:i32[])
                                n3179 = for {
                                N: w4300 -> [_]
                                tunnel: w4305 -> [w4327] mode=indexing
                                tunnel: [w4323] -> w4303 mode=indexing
                                n3180 = Equal To 0?(x=w4327) -> (x = 0?=w4326:bool)
                                n3181 = Select(t="无", s=w4326, f="故障") -> (s? t:f=w4323:string)
                                }
                                n3182 = Insert Into Array(array=w4304, new element=w4303) -> (w4302:string[])  [unwired: 1 in]
                              }
                              n3183 = call "详细故障分解.vi"("名称"=string[] ["上电自检异常(CellV)", "通讯异常(CellV)", "不更新(CellV)", "未校准(CellV)", "保留", "采样线路断路(CellV)", "18b20上电自检异常(T) ", "18b20通讯异常(T)", "18b20传感器丢失(T)", "18b20传感器无号(T)", "18b20温度异常跳变(T)", "18b20信号线对电源短路(T)", "18b20信号线对地短路(T)", "18b20 CRC校验异常(T)", "NTC上电自检异常(T)", "NTC通讯异常(T)", "NTC传感器丢失(T)", "NTC温度异常跳变(T)", "NTC信号线断路(T)", "NTC信号线对电源短(T)", "NTC信号线对地短路(T)", "上电自检异常(Curr)", "参数异常(Curr)", "不更新(Curr)", "未校准(Curr)", "采样线断开(Curr)", "电流零漂异常(Curr)", "传感器反接(Curr)", "读取实时电流故障(Curr)", "平均电流故障(Curr)", "自检异常(iso)", "前端检测电阻损坏(iso)", "不更新(iso)", "未校准(iso)", "上电自检异常(Sumv_in)", "通讯异常(Sumv_in)", "不更新(Sumv_in)", "未校准(Sumv_in)", "上电自检异常(Sumv_out)", "通讯异常(Sumv_out)", "不更新(Sumv_out)", "未校准(Sumv_out)", "系统时钟自检异常(Clock)", "系统时钟未校准(Clock)", "充电均衡模块不能开启", "充电均衡模块不能关闭", "放电均衡模块不能开启", "放电均衡模块不能关闭"], "故障输入口"=w4296) -> ("输出数组"=w4294:string[][])  [unwired: 1 in, 2 out]
                              n3184 = local write "电池故障"(w4294) -> ()
                            }
                            frame 2 {
                              n3185 = for {
                                N: 5 -> [_]
                                tunnel: w4332 -> [w4349]
                                shift-right: [w4336] -> w4330
                                shift-left: string[] [] -> [w4338]
                                i -> [w4334]
                                w4343 = 8 ("索引")
                                w4347 = 2 ("y")
                                n3186 = Multiply(x=w4334, y=w4347) -> (x*y=w4348:i32)
                                n3187 = Array Subset(array=w4349, index=w4348, length=w4347) -> (w4346:u8[])
                                n3188 = Index Array(array=w4346) -> (element #1=w4345:u8, element #2=w4344:u8)  [unwired: 2 in]
                                n3189 = call "二进制解析-8.6.vi"("索引"=w4343, "数值"=w4345) -> ("低位子数组"=w4342:i32[])  [unwired: 1 in, 2 out]
                                n3190 = call "二进制解析-8.6.vi"("索引"=w4343, "数值"=w4344) -> ("低位子数组"=w4341:i32[])  [unwired: 1 in, 2 out]
                                n3191 = Insert Into Array(array=w4342, new element=w4341) -> (w4340:i32[])  [unwired: 1 in]
                                n3192 = case shown="2" w4334 {
                                tunnel: [4 6 5] -> w4335
                                frame 0, Default {
                                }
                                frame 2 {
